vi "Send R_W CMD.vi"(8 "error in":errorcluster, 9 "Input":string, 10 "CMD":string, 11 "PPT in":refnum<class "PPT.lvclass">) -> (0 "error out":errorcluster, 2 "Return":string, 3 "PPT out":refnum<class "PPT.lvclass">)   [LabVIEW 2014, in "PPT Library.lvlib" / "PPT.lvclass"]
doc: "This VI handles communication with the PPTs. The way data sent and retrieved will depend on whether the global channel flag has been set. If this flag has been set, the command will be sent to ALL devices on the network and the VI will read all data from the line until an error is returned on read. If the flag is not set, we will use the current active ID (stored in a DVR) and data will be read only until the termination character (/r) is received."
uses:
  PPT.lvclass
  reusable/Session APIs/Serial/Serial Session.lvclass
panel:
  in  "Global?":bool
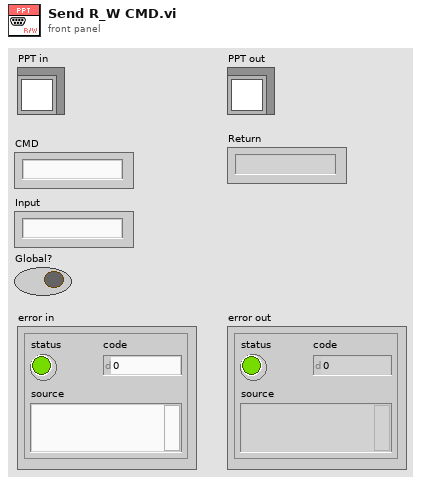
[diagram p1: front panel]
types:
  T1 = typedef "Session - Root.lvclass/Session Handle.ctl" = refnum<data-value>
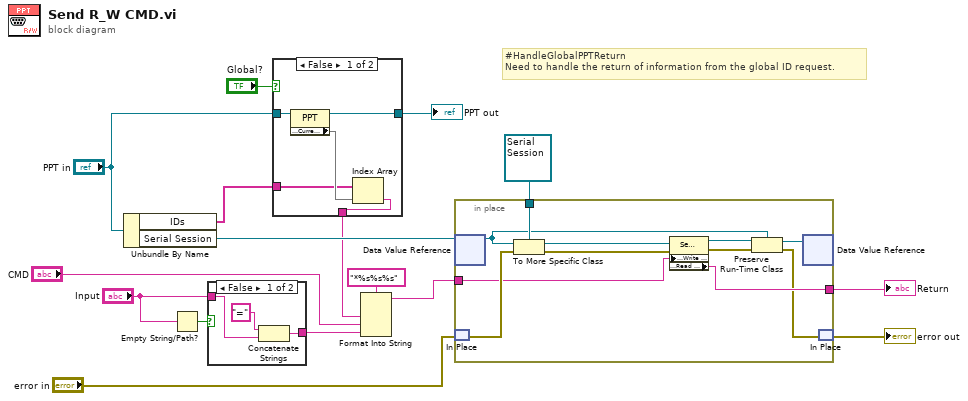
[diagram p0: block diagram]
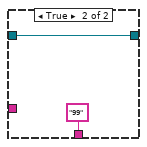
[diagram p2: hidden frame]
diagram:
  # "#HandleGlobalPPTReturn\nNeed to handle the return of information from the global ID request."
  n1 = Unbundle By Name("PPT in") -> ("IDs"=w2:string[], "Serial Session"=w10:T1)
  n2 = Empty String/Path?(string/path="Input") -> (empty?=w8:bool)
  n3 = case shown="False" w8 {
    tunnel: [w17 w20] -> w6
    tunnel: "Input" -> [w19 w20]
    frame False {
      n4 = Concatenate Strings("=" ("string"), w19) -> (w17:string)
    }
    frame True {
    }
  }
  n5 = case shown="False" "Global?" {
    tunnel: "PPT in" -> [w25 w27]
    tunnel: w2 -> [w23 _]
    tunnel: [w22 "99" ("Address")] -> w4
    tunnel: [w21 w27] -> w1
    frame False {
      n6 = property class="PPT"(reference=w25) -> (reference out=w21:refnum<class "PPT.lvclass">, "Utilities:Current ID"=w24)  [unwired: 1 in, 1 out]
      n7 = Index Array(array=w23, index=w24) -> (element=w22:string)
    }
    frame True {
    }
  }
  "PPT out" <- w1
  n8 = Format Into String(format string="*%s%s%s", w4, "CMD", w6) -> (resulting string=w15:string)  [unwired: 2 in, 1 out]
  n9 = in-place {
    in-place-border: refnum<class "Serial Session.lvclass"> refnum ("Serial Session") -> [w37]
    in-place-border: [w34] -> w16
    in-place-border: w15 -> [w28]
    n10 = in-place-dvr #1(w10) -> (w32:refnum<class "Session - Root.lvclass">)  [unwired: 1 out]
    n11 = in-place-match #2("error in") -> (w35:errorcluster)
    n12 = To More Specific Class(target class=w37, reference=w32, error in=w35) -> (specific class reference=w36:refnum<class "Serial Session.lvclass">, error out=w38:errorcluster)
    n13 = property class="Serial Session"(reference=w36, error in=w38, "Public:Write - Asynchronous"=w28) -> (reference out=w33:refnum<class "Serial Session.lvclass">, error out=w30:errorcluster, "Public:Read - Asynchronous"=w34:string)
    n14 = Preserve Run-Time Class(object in=w33, error in=w30, 2:w32) -> (object out=w31:refnum<class "Session - Root.lvclass">, error out=w29:errorcluster)
    n15 = in-place-dvr #1(w31) -> ()  [unwired: 2 out]
    n16 = in-place-match #2(w29) -> (→"error out":errorcluster)
  }
  "Return" <- w16
